vi "Find Index (single).vi"(8 "error in (no error)":errorcluster, 10 "Key":string, 11 "Parameter to Hardware Map in":refnum<class "Parameter to Hardware Map.lvclass">) -> (0 "error out":errorcluster, 1 "Found?":bool, 2 "Index":i32, 3 "Parameter to Hardware Map out":refnum<class "Parameter to Hardware Map.lvclass">)   [LabVIEW 2020, in "RxnRover.lvlib" / "Parameter to Hardware Map.lvclass"]
doc: "Return the index from the map specified by the given key."
uses:
  Parameter to Hardware Map.lvclass
  Parameter to Hardware Map.lvclass/Parameter to Hardware Map.ctl
  Controller/Generic Plugin.lvclass
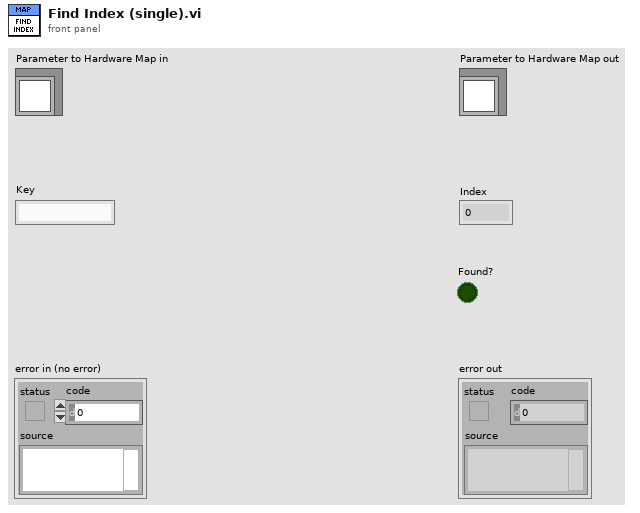
[diagram p1: front panel]
types:
  T1 = typedef "RxnRover.lvlib/Parameter to Hardware Map.lvclass/Pair.ctl" = cluster{"key":string, "values":refnum<class "Generic Plugin.lvclass">[]}
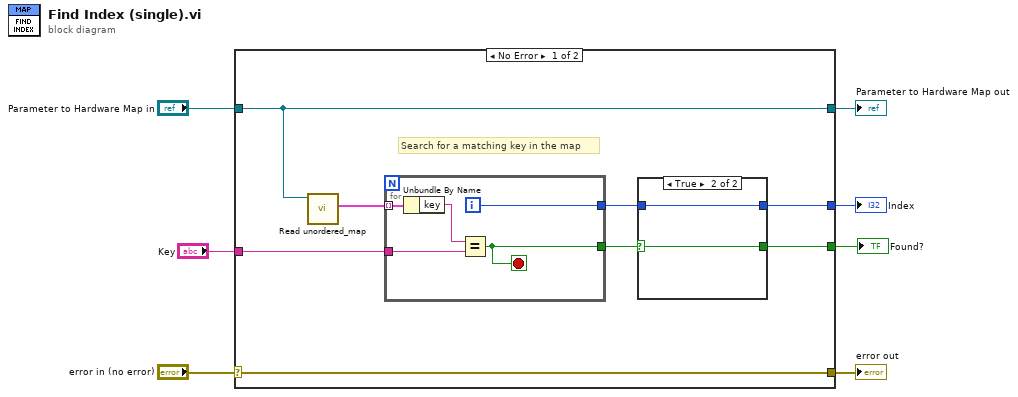
[diagram p0: block diagram]
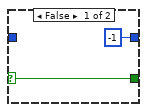
[diagram p2: hidden frame]
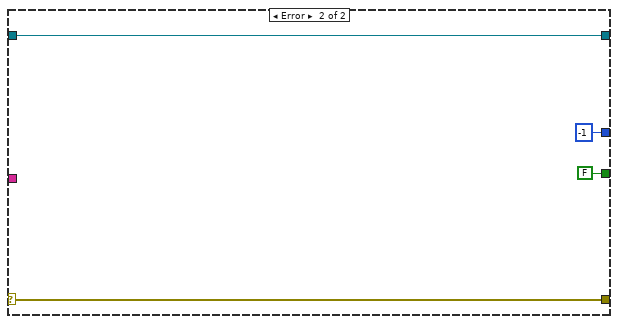
[diagram p3: hidden frame]
diagram:
  n1 = case shown="No Error" "error in (no error)" {
    selector: "error in (no error)" -> [w15 w28]
    tunnel: [w15 w28] -> w6
    tunnel: [w14 w27] -> w4
    tunnel: "Parameter to Hardware Map in" -> [w14 w27]
    tunnel: "Key" -> [w12 _]
    tunnel: [w9 -1] -> w2
    tunnel: [w8 FALSE] -> w1
    frame No Error {
      # "Search for a matching key in the map"
      n2 = call "Read unordered_map.vi"("Parameter to Hardware Map in"=w14) -> ("unordered_map"=w13:T1[])  [unwired: 8 in, 2 out]
      n3 = for {
        tunnel: w13 -> [w24] mode=indexing
        tunnel: w12 -> [w22]
        tunnel: [w21] -> w11
        tunnel: [w20] -> w10
        i -> [w20]
        stop <- w21 stop-if-true
        n4 = Unbundle By Name(w24) -> ("key"=w23:string)
        n5 = Equal?(x=w23, y=w22) -> (x = y?=w21:bool)
      }
      n6 = case shown="True" w11 {
        selector: w11 -> [w16 w18]
        tunnel: w10 -> [_ w19]
        tunnel: [-1 w19] -> w9
        tunnel: [w16 w18] -> w8
        frame False {
        }
        frame True {
        }
      }
    }
    frame Error {
    }
  }
  "error out" <- w6
  "Parameter to Hardware Map out" <- w4
  "Index" <- w2
  "Found?" <- w1
